vi "Welcome To Demo Sandbox.vi"() -> ()   [LabVIEW 2019]
panel:
  out "appended array":i32[](array[numeric])
  in  "next":bool
  in  "stop":bool
  out "Numeric 3":dbl
  out "Numeric 2":dbl
  out "Numeric":dbl
  out "2D Picture 3":picture
  out "2D Picture 2":picture
  out "2D Picture":picture
  out "size(s) 2":i32
  out "size(s)":i32
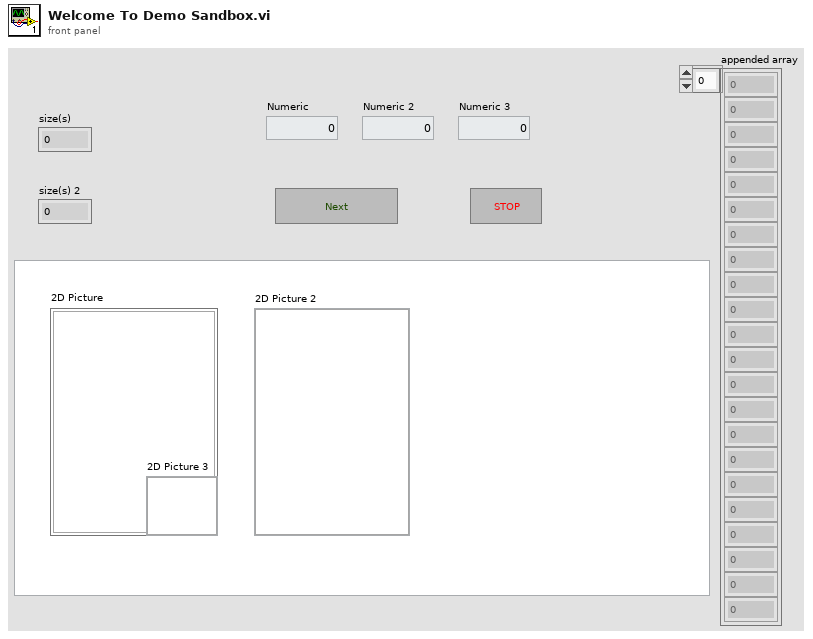
[diagram p1: front panel]
types:
  T1 = typedef "imagedata.ctl" = cluster{"image type":i32, "image depth":i32, "image":u8[], "mask":u8[], "colors":u32[], "Rectangle":cluster{"left":i16, "top":i16, "right":i16, "bottom":i16}}
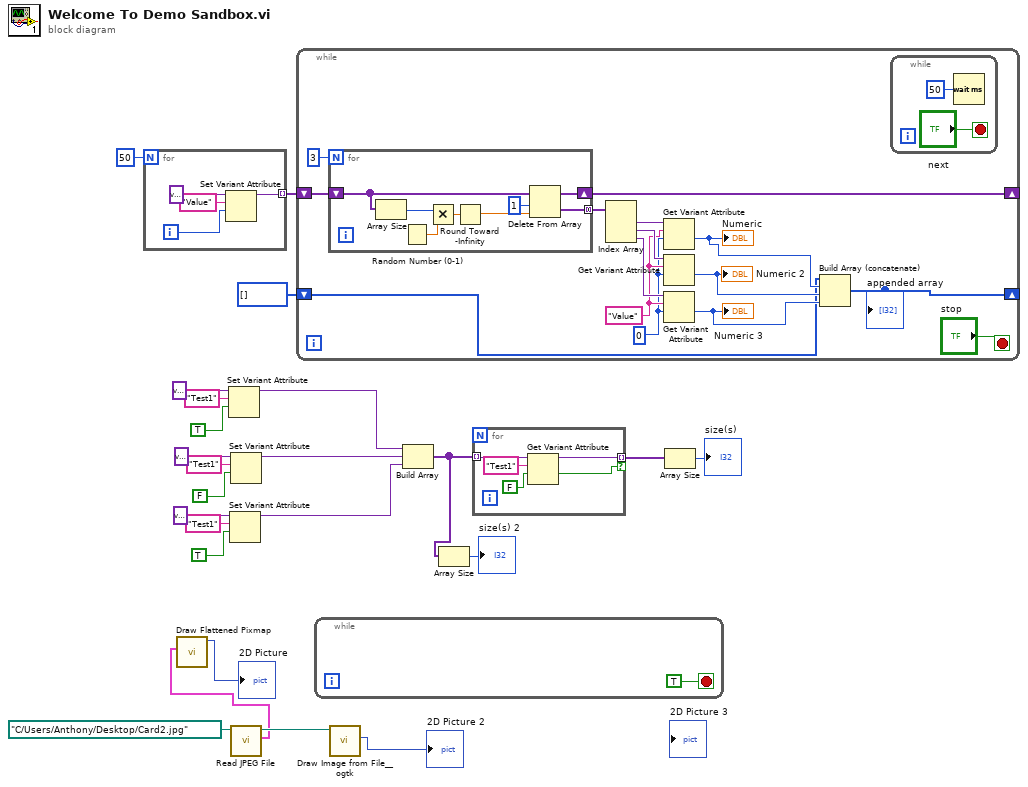
[diagram p0: block diagram]
diagram:
  n1 = for {
    N: 50 -> [_]
    tunnel: [w25] -> w2 mode=indexing
    i -> [w26]
    n2 = Set Variant Attribute(Variant=variant, name="Value", value=w26) -> (Variant out=w25:variant)  [unwired: 1 in, 2 out]
  }
  n3 = Set Variant Attribute(Variant=variant, name="Test1", value=TRUE) -> (Variant out=w15:variant)  [unwired: 1 in, 2 out]
  n4 = Set Variant Attribute(Variant=variant, name="Test1", value=TRUE) -> (Variant out=w13:variant)  [unwired: 1 in, 2 out]
  n5 = Set Variant Attribute(Variant=variant, name="Test1", value=FALSE) -> (Variant out=w14:variant)  [unwired: 1 in, 2 out]
  n6 = call <vilib>:"Read JPEG File.vi"("path to JPEG file"=path "C:/Users/Anthony/Desktop/Card2.jpg") -> ("image data"=w5:T1, "path"=w6:path)  [unwired: 8 in, 1 out]
  n7 = call <vilib>:"Draw Flattened Pixmap.vi"("image data"=w5) -> ("new picture"=→"2D Picture":picture)  [unwired: 8 in]
  n8 = while {
    shift-right: [w31] -> _
    shift-left: i32[] [] -> [w30]
    shift-right: [w29] -> _
    shift-left: w2 -> [w42]
    stop <- "stop" stop-if-true
    w36 = 0
    w37 = "Value" ("name")
    n9 = for {
      N: 3 -> [_]
      shift-right: [w47] -> w29
      shift-left: w42 -> [w50]
      tunnel: [w46] -> w41 mode=concatenating
      n10 = Array Size(array=w50) -> (size(s)=w52:i32)
      n11 = Random Number (0-1)() -> (number: 0 to 1=w53:dbl)
      n12 = Multiply(x=w52, y=w53) -> (x*y=w51:dbl)
      n13 = Round Toward -Infinity(1:w51) -> (0:w48:dbl)
      n14 = Delete From Array(array=w50, length=1, index=w48) -> (deleted portion=w46:variant[], array with subset deleted=w47:variant[])
    }
    n15 = Index Array(array=w41) -> (element #1=w40:variant, element #2=w39:variant, element #3=w38:variant)  [unwired: 3 in]
    n16 = Get Variant Attribute(Variant=w40, name=w37, default value (empty Variant)=w36) -> (value=w34:i32)  [unwired: 1 in, 3 out]
    "Numeric" <- w34
    n17 = Get Variant Attribute(Variant=w39, name=w37, default value (empty Variant)=w36) -> (value=w33:i32)  [unwired: 1 in, 3 out]
    "Numeric 2" <- w33
    n18 = Get Variant Attribute(Variant=w38, name=w37, default value (empty Variant)=w36) -> (value=w32:i32)  [unwired: 1 in, 3 out]
    "Numeric 3" <- w32
    n19 = Build Array (concatenate)(w30, w34, w33, w32) -> (w31:i32[])
    "appended array" <- w31
    n20 = while {
      stop <- "next" stop-if-true
      n21 = Wait (ms)(milliseconds to wait=u32 50) -> ()  [unwired: 1 out]
    }
  }
  n22 = while {
    stop <- TRUE stop-if-true
  }
  n23 = call <userlib>:"Draw Image from File__ogtk.vi"("path to image file"=w6) -> ("new picture"=→"2D Picture 2":picture)  [unwired: 7 in, 3 out]
  n24 = Build Array(w15, w14, w13) -> (w9:variant[])
  n25 = Array Size(array=w9) -> (size(s)=→"size(s) 2":i32)
  n26 = for {
    tunnel: w9 -> [w59] mode=indexing
    tunnel: [w56] -> w12 mode=indexing if=w55
    n27 = Get Variant Attribute(Variant=w59, name="Test1", default value (empty Variant)=FALSE) -> (duplicate Variant=w56:variant, value=w55:bool)  [unwired: 1 in, 2 out]
  }
  n28 = Array Size(array=w12) -> (size(s)=→"size(s)":i32)
